vi "extract TTL timing data.vi"(9 "threshold":dbl=1.0 format="%#_13g", 11 "Waveform":waveform(dbl)) -> (3 "x+y":timestamp[](array[timestamp]))   [LabVIEW 2025]
uses:
  <vilib>/Analysis/NI_AALPro.lvlib
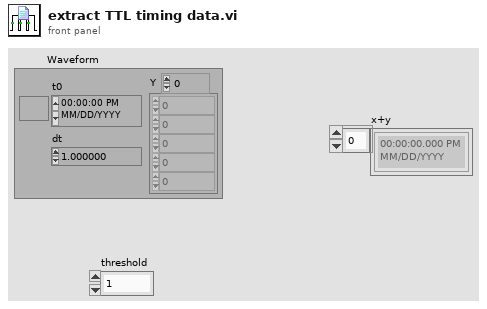
[diagram p1: front panel]
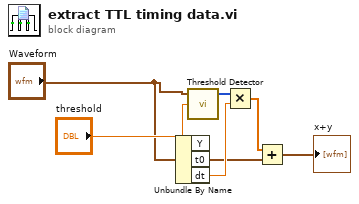
[diagram p0: block diagram]
diagram:
  n1 = Unbundle By Name("Waveform") -> ("t0"=w3:timestamp, "dt"=w6:dbl)  [unwired: 1 out]
  n2 = call <vilib>:"Threshold Detector.vi"("threshold"="threshold", "X"="Waveform") -> ("Indices"=w7:i32[])  [unwired: 1 in, 2 out]
  n3 = Multiply(x=w7, y=w6) -> (x*y=w5:dbl[])
  n4 = Add(x=w5, y=w3) -> (x+y=→"x+y":timestamp[])
